vi "Cargo Intake.vi"   [LabVIEW 2018]
uses:
  <vilib>/Rock Robotics/WPI/Solenoid/WPI_SolenoidChannel.ctl
  <vilib>/Rock Robotics/SystemInterfaces/DIO/FPGA_DIOChannel.ctl
  <vilib>/Rock Robotics/WPI/ThirdParty/Phoenix-LabVIEW/Motor Controller/Controls/CTRE_Phoenix_MotorControl_ControlMode.ctl
  <vilib>/Rock Robotics/WPI/Solenoid/WPI_SolenoidValue.ctl
  Cargo Intake Global.vi
  <vilib>/Rock Robotics/WPI/Solenoid/WPI_SolenoidOpenDouble.vi
  <vilib>/Rock Robotics/WPI/Counter/WPI_CounterDigitalInputToDigitalSource.vi
  <vilib>/Rock Robotics/WPI/Switch/WPI_SwitchOpenLimit.vi
  Controllers/Manipulator Controlller/Manipulator Controller Global.vi
  Sensors/Sensors Global.vi
  Times/Times Global.vi
  <vilib>/Rock Robotics/WPI/Solenoid/WPI_SolenoidSetEnum.vi
types:
  T1 = typedef "FPGA_DIOChannel.ctl" = enum8{"DIO 0", "DIO 1", "DIO 2", "DIO 3", "DIO 4", "DIO 5", "DIO 6", "DIO 7", "DIO 8", "DIO 9", "DIO MXP 0", "DIO MXP 1", "DIO MXP 2", "DIO MXP 3", "DIO MXP 4", "DIO MXP 5", "DIO MXP 6", "DIO MXP 7", "DIO MXP 8", "DIO MXP 9", "DIO MXP 10", "DIO MXP 11", "DIO MXP 12", "DIO MXP 13", "DIO MXP 14", "DIO MXP 15", "SPI Port CS1", "SPI Port CS2", "SPI Port CS3", "SPI Port MISO", "SPI Port MOSI", "Invalid"}
  T2 = typedef "WPI_SolenoidChannel.ctl" = enum8{"Solenoid 0", "Solenoid 1", "Solenoid 2", "Solenoid 3", "Solenoid 4", "Solenoid 5", "Solenoid 6", "Solenoid 7", "Invalid"}
  T3 = enum16{"Full Manual Control", "Manual Control", "Automated Control"}
  T4 = typedef "WPI_SolenoidValue.ctl" = enum16{"Off", "On", "Forward", "Reverse"}
  T5 = typedef "WPI_DigitalInputDevRef.ctl" = cluster{"DevStatus":errorcluster, "DIO Channel":T1}
  T6 = typedef "FPGA_CounterEncoderSourceConvertionLVSourceType.ctl" = cluster{"DevStatus":errorcluster, "AnalogTriggerMode?":bool, "DigitalMode":cluster{"DIO Channel":T7}, "AnalogTriggerMode":cluster{"AnalogTriggerIndex":T8, "OutputType":T9}}
  T7 = typedef "FPGA_DIODigitalSourceChannel.ctl" = enum8{"DIO 0", "DIO 1", "DIO 2", "DIO 3", "DIO 4", "DIO 5", "DIO 6", "DIO 7", "DIO 8", "DIO 9", "DIO MXP 0", "DIO MXP 1", "DIO MXP 2", "DIO MXP 3", "DIO MXP 4", "DIO MXP 5", "DIO MXP 6", "DIO MXP 7", "DIO MXP 8", "DIO MXP 9", "DIO MXP 10", "DIO MXP 11", "DIO MXP 12", "DIO MXP 13", "DIO MXP 14", "DIO MXP 15", "SPI Port CS1", "SPI Port CS2", "SPI Port CS3", "SPI Port MISO", "SPI Port MOSI", "Disabled"}
  T8 = typedef "FPGA_AnalogTriggerIndex.ctl" = enum8{"Trig 0", "Trig 1", "Trig 2", "Trig 3", "Trig 4", "Trig 5", "Trig 6", "Trig 7", "Invalid"}
  T9 = typedef "FPGA_AnalogTriggerOutType.ctl" = enum16{"InWindow", "TriggerState", "Rising", "Falling"}
  T10 = typedef "WPI_EncoderDevRef.ctl" = cluster{"DevStatus":errorcluster, "EncoderIndex":T11, "CounterIndex":T12, "DistancePerCount":dbl, "Decoding Type":T13}
  T11 = typedef "FPGA_EncoderIdx.ctl" = enum8{"Enc 0", "Enc 1", "Enc 2", "Enc 3", "Enc 4", "Enc 5", "Enc 6", "Enc 7", "Invalid"}
  T12 = typedef "FPGA_CounterCtrSystemIndex.ctl" = enum8{"Ctr 0", "Ctr 1", "Ctr 2", "Ctr 3", "Ctr 4", "Ctr 5", "Ctr 6", "Ctr 7", "Invalid"}
  T13 = typedef "WPI_EncoderType.ctl" = enum16{"1x", "2x", "4x"}
  T14 = typedef "WPI_SolenoidDevRef.ctl" = cluster{"DevStatus":errorcluster, "Pneumatics Control Module":u8, "Forward Solenoid Channel":T2, "Reverse Solenoid Channel":T2}
  T15 = typedef "WPI_SwitchDevRef.ctl" = cluster{"DevStatus":errorcluster, "DIO Channel":T1, "CntIndex":T12, "Normally Closed":bool}
  T16 = typedef "WPI_MotorControlDeviceRef.ctl" = cluster{"DeviceStatus":errorcluster, "Type":T17, "PWM":cluster{"PWM Channel":T18, "DeadBand":T19}, "CAN":cluster{"Device Number":u8, "SetOutput VI Ref":variant, "GetOutput VI Ref":variant, "Enable VI Ref":variant, "Disable VI Ref":variant, "Data":variant}, "Invert":bool, "DIO PWM":cluster{"PWM \"Enable\" Channel":T18, "DIOChannel":T1, "PWM Rate":dbl}}
  T17 = typedef "WPI_MotorControlType.ctl" = enum16{"PWM", "CAN", "DIO PWM"}
  T18 = typedef "FPGA_DIOPWMChannel.ctl" = enum8{"PWM 0", "PWM 1", "PWM 2", "PWM 3", "PWM 4", "PWM 5", "PWM 6", "PWM 7", "PWM 8", "PWM 9", "PWM MXP 0", "PWM MXP 1", "PWM MXP 2", "PWM MXP 3", "PWM MXP 4", "PWM MXP 5", "PWM MXP 6", "PWM MXP 7", "PWM MXP 8", "PWM MXP 9", "Invalid"}
  T19 = typedef "WPI_PWMDeadband.ctl" = cluster{"Name":string, "maxPositivePwm":i32, "minPositivePwm":i32, "centerPwm":i32, "maxNegativePwm":i32, "minNegativePwm":i32, "angularRange":u16}
  T20 = typedef "CTRE_Phoenix_MotorControl_ControlMode.ctl" = u16
  T21 = typedef "Control 1.ctl" = dbl
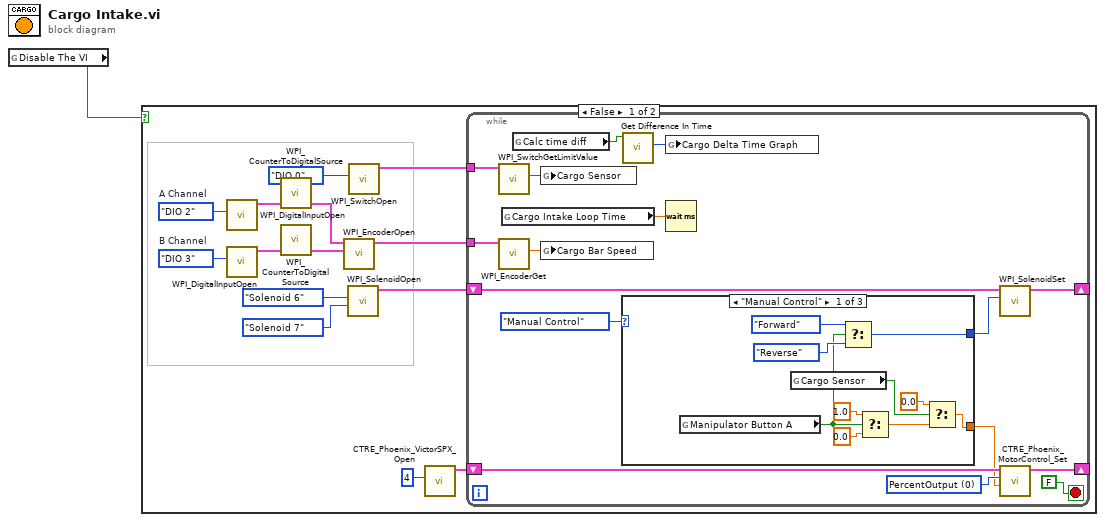
[diagram p0: block diagram]
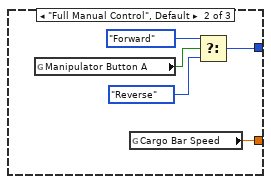
[diagram p2: hidden frame]
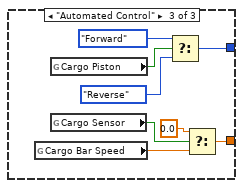
[diagram p3: hidden frame]
diagram:
  n1 = global read "Cargo Intake Global.vi" "Disable The VI"() -> (w1:bool)
  n2 = case shown="False" w1 {
    frame False {
      w10 = FPGA_DIOChannel."DIO 3"  # B Channel
      w9 = FPGA_DIOChannel."DIO 2"  # A Channel
      n3 = call <vilib>:"WPI_DigitalInputOpen.vi"("DIO Channel"=w9) -> ("DigitalInputDevRef"=w6:T5)  [unwired: 1 in, 9 out]
      n4 = call <vilib>:"WPI_DigitalInputOpen.vi"("DIO Channel"=w10) -> ("DigitalInputDevRef"=w7:T5)  [unwired: 1 in, 9 out]
      n5 = call-poly <vilib>:"WPI_CounterToDigitalSource.vi"("DigitalInputDevRef"=w6) -> ("Digital Source"=w5:T6)  [unwired: 6 out]
      n6 = call-poly <vilib>:"WPI_CounterToDigitalSource.vi"("DigitalInputDevRef"=w7) -> ("Digital Source"=w8:T6)  [unwired: 6 out]
      n7 = call <vilib>:"WPI_EncoderOpen.vi"("BSource"=w8, "ASource"=w5) -> ("EncoderDevRef"=w4:T10)  [unwired: 6 in, 3 out]
      n8 = call-poly <vilib>:"WPI_SolenoidOpen.vi"("Reverse Solenoid Channel"=WPI_SolenoidChannel."Solenoid 7" ("Solenoid Channel"), "Forward Solenoid Channel"=WPI_SolenoidChannel."Solenoid 6" ("Solenoid Channel")) -> ("SolenoidDevRef"=w11:T14)  [unwired: 8 in, 1 out]
      n9 = call-poly <vilib>:"WPI_SwitchOpen.vi"("DIO Channel"=FPGA_DIOChannel."DIO 0") -> ("SwitchDevRef"=w3:T15)  [unwired: 9 in, 1 out]
      n10 = call <vilib>:"CTRE_Phoenix_VictorSPX_Open.vi"("Device Number"=u8 4) -> ("CAN Talon SRX Ref"=w14:T16)  [unwired: 9 in, 1 out]
      n11 = while {
        shift-right: [w26] -> _
        shift-left: w14 -> [w24]
        shift-right: [w22] -> _
        shift-left: w11 -> [w21]
        tunnel: w4 -> [w19]
        tunnel: w3 -> [w17]
        stop <- FALSE stop-if-true
        w25 = T20 0 items=["PercentOutput"=0, "Position"=1, "Velocity"=2, "Current"=3, "Follower"=5, "MotionProfile"=6, "MotionMagic"=7, "MotionProfileArc"=10, "Disabled"=15] ("Control Mode")
        n12 = call <vilib>:"WPI_SwitchGetLimitValue.vi"("SwitchDevRef"=w17) -> ("Switch Pressed"=w16:bool)  [unwired: 8 in, 2 out]
        n13 = call <vilib>:"WPI_EncoderGet.vi"("EncoderDevRef"=w19) -> ("Distance"=w18:dbl)  [unwired: 5 in, 5 out]
        n14 = global read "Times Global.vi" "Cargo Intake Loop Time"() -> (w31:T21)
        n15 = global read "Cargo Intake Global.vi" "Calc time diff"() -> (w29:bool)
        n16 = global write "Cargo Intake Global.vi" "Cargo Sensor"(w16) -> ()
        n17 = global write "Cargo Intake Global.vi" "Cargo Bar Speed"(w18) -> ()
        n18 = case shown="\"Manual Control\"" T3."Manual Control" ("Cargo Intake Mode") {
          tunnel: [w39 w46 w54] -> w23
          tunnel: [w34 w42 w49] -> w20
          frame "Manual Control" {
            n19 = global read "Manipulator Controller Global.vi" "Manipulator Button A"() -> (w33:bool)
            n20 = global read "Sensors Global.vi" "Cargo Sensor"() -> (w32:bool)
            n21 = Select(t=WPI_SolenoidValue."Forward" ("Value"), s=w33, f=WPI_SolenoidValue."Reverse" ("Value")) -> (s? t:f=w34:T4)
            n22 = Select(t=1.0, s=w33, f=0.0 ("t")) -> (s? t:f=w41:dbl)
            n23 = Select(t=0.0, s=w32, f=w41) -> (s? t:f=w39:dbl)
          }
          frame "Full Manual Control", Default {
            n24 = global read "Manipulator Controller Global.vi" "Manipulator Button A"() -> (w43:bool)
            n25 = global read "Cargo Intake Global.vi" "Cargo Bar Speed"() -> (w46:dbl)
            n26 = Select(t=WPI_SolenoidValue."Forward" ("Value"), s=w43, f=WPI_SolenoidValue."Reverse" ("Value")) -> (s? t:f=w42:T4)
          }
          frame "Automated Control" {
            n27 = global read "Cargo Intake Global.vi" "Cargo Bar Speed"() -> (w52:dbl)
            n28 = global read "Cargo Intake Global.vi" "Cargo Piston"() -> (w48:bool)
            n29 = global read "Sensors Global.vi" "Cargo Sensor"() -> (w47:bool)
            n30 = Select(t=WPI_SolenoidValue."Forward" ("Value"), s=w48, f=WPI_SolenoidValue."Reverse" ("Value")) -> (s? t:f=w49:T4)
            n31 = Select(t=0.0, s=w47, f=w52) -> (s? t:f=w54:dbl)
          }
        }
        n32 = call "Get Difference In Time.vi"("Calculate Time Difference"=w29) -> ("Delta Time over Time"=w27:u32)  [unwired: 9 in, 1 out]
        n33 = global write "Times Global.vi" "Cargo Delta Time Graph"(w27) -> ()
        n34 = Wait (ms)(milliseconds to wait=w31) -> ()  [unwired: 1 out]
        n35 = call-poly <vilib>:"WPI_SolenoidSet.vi"("Value"=w20, "SolenoidDevRef"=w21) -> ("SolenoidDevRef"=w22:T14)  [unwired: 8 in, 1 out]
        n36 = call <vilib>:"CTRE_Phoenix_MotorControl_Set.vi"("Output"=w23, "Control Mode"=w25, "PhoenixMotorControlDevRef"=w24) -> ("PhoenixMotorControlDevRef"=w26:T16)  [unwired: 7 in, 1 out]
      }
    }
    frame True {
    }
  }
